vi "SEM Scan Parameter Coerce.vi"(6 "X full scale (V)":dbl, 7 "AI upper limit":dbl=100000000.0, 8 "SEM Status":T3={"AO SampClk.MaxRate"=100000000.0, "AI SampClk.MaxRate"=100000000.0, "AO rate"=10000000.0, "Scan speed"=4, "Detector #"=1, "X min (V)"=-10.0, "X max (V)"=10.0, "X min index"=0, "X max index"=1023, "AO multiline"=512, "Decimating factor"=2, "AvailSampPerChan"=0, "AO scan line"=0, "Total pixels recorded"=0, "Lines scanned"=0, "Scan time (m)"=0.0, "Scan time (s)"=4.15236096, "Remaining time (m)"=0, "Remaining time (s)"=0, "Specimen I (nA)"=0.0, "Frame"=1, "X tile"=1, "Y tile"=1} {"Frame" min=1 step=1; "Y tile" min=1; "X tile" min=1; "Specimen I (nA)" format="%.2g"; "AvailSampPerChan" scale=0.0..32000000.0; "Scan time (s)" format="%.3f"; "Total pixels recorded" scale=-1.0..37748736.0; "Scan speed" scale=1.0..15.0; "AO rate" format="%#_3e"}, 9 "SEM Options":T2={"GetInfo"=TRUE, "Set Det A para"=TRUE, "Set WD"=FALSE, "Set Mag"=TRUE, "Set stig"=FALSE, "Set aln"=FALSE, "Display"=TRUE, "Save"=TRUE, "8-bit"=TRUE, "Detector A"=TRUE, "Detector B"=FALSE, "Detector C"=FALSE, "Detector D"=FALSE, "Inverse A"=FALSE, "Inverse B"=FALSE, "Inverse C"=FALSE, "Inverse D"=FALSE, "Inverse PNG"=TRUE, "Freeze"=TRUE, "PNG only"=FALSE, "Upload"=FALSE, "Delete after upload"=FALSE}, 10 "SEM Scan Parameters":T1={"X size (um)"=20.0, "Y size (um)"=20.0, "X center (um)"=0.0, "Y center (um)"=0.0, "X size (V)"=6.190428211586902, "X size auto"=TRUE, "X stig"=[[0.0]], "Y stig"=[[0.0]], "X aln"=[[0.0]], "Y aln"=[[0.0]], "Scan rate (Hz)"=10000000, "Oversampling"=5, "Oversampling auto"=TRUE, "Frame line rampdown ratio"=0.1, "Pixel size (nm)"=10.0, "WD (mm)"=[[3.0]], "X tiles"=1, "Y tiles"=1, "Overlap (um)"=1.0, "Interlaced"=TRUE, "dX (um)"=[0.0], "dY (um)"=[0.0], "Frames"=1} {"dY (um)" format="%.1f"; "dX (um)" format="%.1f"; "Frames" min=1 step=1; "WD (mm)" format="%.1f"; "Y aln" format="%.1f"; "X aln" format="%.1f"; "Y stig" format="%.1f"; "X stig" format="%.1f"; "Overlap (um)" min=0; "Y tiles" min=1; "X tiles" min=1; "X size (um)" format="%.2f"; "Y size (um)" format="%.2f"; "Frame line rampdown ratio" min=0 max=1 step=0.05 format="%.2g"; "X center (um)" step=1.0 format="%.2f"; "Y center (um)" step=1.0 format="%.2f"; "X size (V)" format="%_4g"; "Scan rate (Hz)" max=4000000 step=100000 format="%.2e"}, 11 "Hardware Configuration":T4={"SEM X coil"="SEM-X", "SEM Y coil"="SEM-Y", "FIB X coil"="FIB/ao0", "FIB Y coil"="FIB/ao1", "FIB Detector"="FIB/ai1", "SEM Detectors"="Detectors", "Det min (V)"=-10.0, "Det max (V)"=10.0, "Eanable COM"=TRUE, "COM port"="COM1", "FIB Beam blank"="FIB/port0/line0", "FIB Ext Scan"="FIB/port0/line1", "Det. FIB-NI auto switch"="FIB/port0/line2", "Post #1up"="Log/ao0", "Post #1down"="Log/ao1", "Post #2up"="Log/ao2", "Post #2down"="Log/ao3", "Machine Type"=0, "FIB Faraday Cup"="FIB/ai3", "Configuration file"=path "D:/3D FIB-SEM Files/Feiss.ini", "SEM Max FOV (um)"=198.5, "Machine ID"="Feiss2/Merlin-4238", "Save config file"=FALSE, "Temperature port"="COM3", "Brightness A"=30.0, "Contrast A"=25.0, "Detector B name"="ESB", "Brightness B"=50.0, "Contrast B"=30.0, "Logging Device"="Log"} {"Machine Type" items=["Feiss", "NVision", "Jeiss"]}) -> (1 "Coerced SEM Scan Parameters":T1={"X size (um)"=20.0, "Y size (um)"=20.0, "X center (um)"=0.0, "Y center (um)"=0.0, "X size (V)"=6.190428211586902, "X size auto"=TRUE, "X stig"=[[0.0]], "Y stig"=[[0.0]], "X aln"=[[0.0]], "Y aln"=[[0.0]], "Scan rate (Hz)"=10000000, "Oversampling"=5, "Oversampling auto"=TRUE, "Frame line rampdown ratio"=0.1, "Pixel size (nm)"=10.0, "WD (mm)"=[[3.0]], "X tiles"=1, "Y tiles"=1, "Overlap (um)"=1.0, "Interlaced"=TRUE, "dX (um)"=[0.0], "dY (um)"=[0.0], "Frames"=1} {"dY (um)" format="%.1f"; "dX (um)" format="%.1f"; "Frames" min=1 step=1; "WD (mm)" format="%.1f"; "Y aln" format="%.1f"; "X aln" format="%.1f"; "Y stig" format="%.1f"; "X stig" format="%.1f"; "Overlap (um)" min=0; "Y tiles" min=1; "X tiles" min=1; "X size (um)" format="%.2f"; "Y size (um)" format="%.2f"; "Frame line rampdown ratio" min=0 max=1 step=0.05 format="%.2g"; "X center (um)" step=1.0 format="%.2f"; "Y center (um)" step=1.0 format="%.2f"; "X size (V)" format="%_4g"; "Scan rate (Hz)" max=4000000 step=100000 format="%.2e"}, 2 "SEM FOV":dbl=198.5, 3 "Detector number":i16)   [LabVIEW 2018]
panel:
  # "Det"
  # "after"
  # "Hz"
  # "Scanning time"
  # "m"
  # "s"
  # "Remaining time"
  # "m"
  # "s"
  # "Detector"
  # "Brightness & Contrast (%)"
  # "A       InLens"
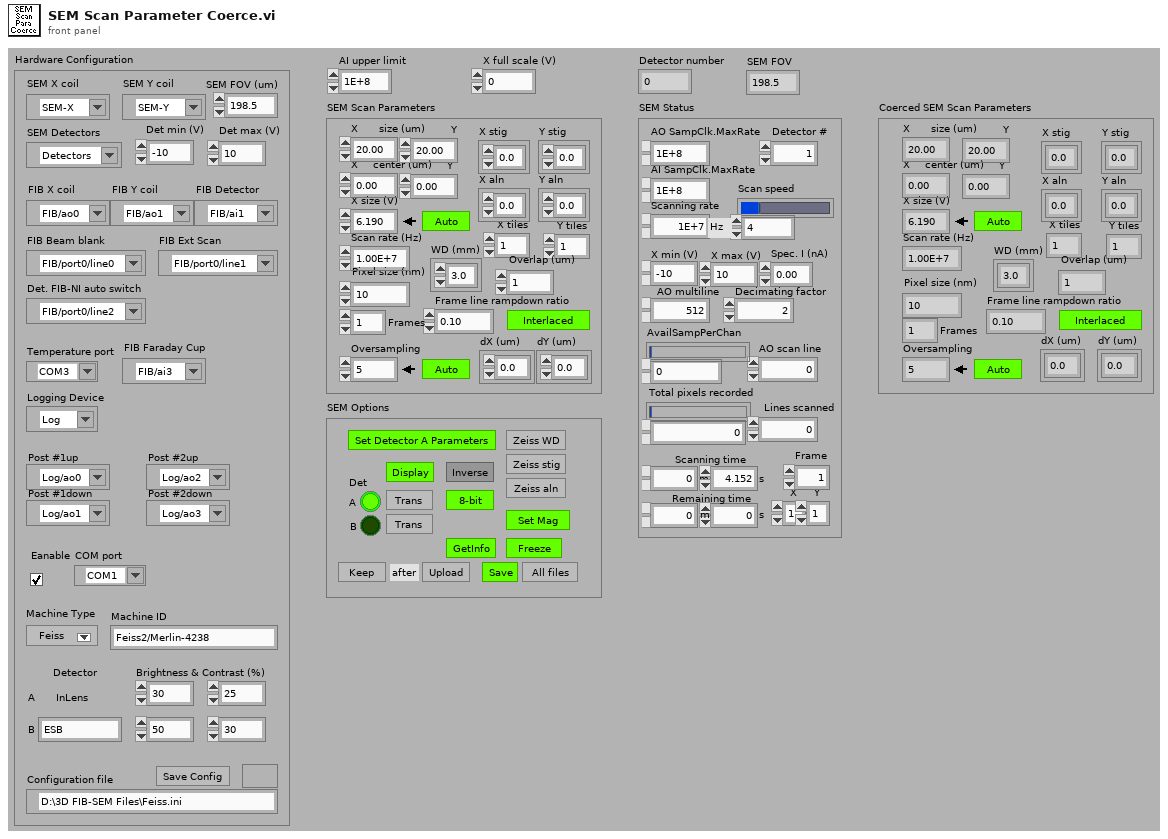
[diagram p1: front panel]
types:
  T1 = cluster{"X size (um)":sgl, "Y size (um)":sgl, "X center (um)":dbl, "Y center (um)":dbl, "X size (V)":dbl, "X size auto":bool, "X stig":sgl[][], "Y stig":sgl[][], "X aln":sgl[][], "Y aln":sgl[][], "Scan rate (Hz)":u32, "Oversampling":u32, "Oversampling auto":bool, "Frame line rampdown ratio":sgl, "Pixel size (nm)":sgl, "WD (mm)":sgl[][], "X tiles":u8, "Y tiles":u8, "Overlap (um)":sgl, "Interlaced":bool, "dX (um)":sgl[], "dY (um)":sgl[], "Frames":u8}
  T2 = cluster{"GetInfo":bool, "Set Det A para":bool, "Set WD":bool, "Set Mag":bool, "Set stig":bool, "Set aln":bool, "Display":bool, "Save":bool, "8-bit":bool, "Detector A":bool, "Detector B":bool, "Detector C":bool, "Detector D":bool, "Inverse A":bool, "Inverse B":bool, "Inverse C":bool, "Inverse D":bool, "Inverse PNG":bool, "Freeze":bool, "PNG only":bool, "Upload":bool, "Delete after upload":bool}
  T3 = cluster{"AO SampClk.MaxRate":dbl, "AI SampClk.MaxRate":dbl, "AO rate":dbl, "Scan speed":u8, "Detector #":u8, "X min (V)":dbl, "X max (V)":dbl, "X min index":i32, "X max index":i32, "AO multiline":u32, "Decimating factor":u16, "AvailSampPerChan":u32, "AO scan line":u32, "Total pixels recorded":i32, "Lines scanned":i32, "Scan time (m)":dbl, "Scan time (s)":dbl, "Remaining time (m)":u16, "Remaining time (s)":u8, "Specimen I (nA)":sgl, "Frame":u8, "X tile":u8, "Y tile":u8}
  T4 = cluster{"SEM X coil":refnum<k15>, "SEM Y coil":refnum<k15>, "FIB X coil":tag, "FIB Y coil":tag, "FIB Detector":tag, "SEM Detectors":refnum<k15>, "Det min (V)":dbl, "Det max (V)":dbl, "Eanable COM":bool, "COM port":refnum<visa-resource-name>, "FIB Beam blank":tag, "FIB Ext Scan":tag, "Det. FIB-NI auto switch":tag, "Post #1up":tag, "Post #1down":tag, "Post #2up":tag, "Post #2down":tag, "Machine Type":u8, "FIB Faraday Cup":tag, "Configuration file":path, "SEM Max FOV (um)":dbl, "Machine ID":string, "Save config file":bool, "Temperature port":refnum<visa-resource-name>, "Brightness A":dbl, "Contrast A":dbl, "Detector B name":string, "Brightness B":dbl, "Contrast B":dbl, "Logging Device":tag}
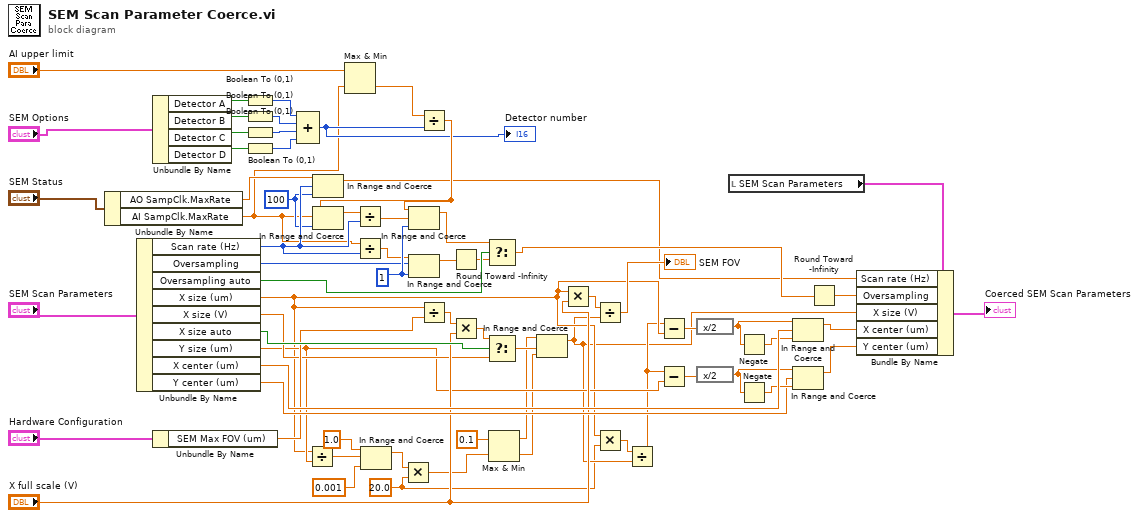
[diagram p0: block diagram]
diagram:
  w1 = 20.0 ("upper limit")
  w51 = u8 1 ("lower limit")
  w43 = u32 100 ("lower limit")
  n1 = Unbundle By Name("SEM Status") -> ("AO SampClk.MaxRate"=w39:dbl, "AI SampClk.MaxRate"=w24:dbl)
  n2 = Unbundle By Name("SEM Scan Parameters") -> ("Scan rate (Hz)"=w46:u32, "Oversampling"=w38:u32, "Oversampling auto"=w45:bool, "X size (um)"=w4:sgl, "X size (V)"=w15:dbl, "X size auto"=w54:bool, "Y size (um)"=w11:sgl, "X center (um)"=w67:dbl, "Y center (um)"=w57:dbl)
  n3 = Unbundle By Name("SEM Options") -> ("Detector A"=w30:bool, "Detector B"=w34:bool, "Detector C"=w35:bool, "Detector D"=w36:bool)
  n4 = Unbundle By Name("Hardware Configuration") -> ("SEM Max FOV (um)"=w53:dbl)
  n5 = Boolean To (0,1)(Boolean=w30) -> (0, 1=w29:i16)
  n6 = Boolean To (0,1)(Boolean=w34) -> (0, 1=w28:i16)
  n7 = Boolean To (0,1)(Boolean=w35) -> (0, 1=w33:i16)
  n8 = Boolean To (0,1)(Boolean=w36) -> (0, 1=w32:i16)
  n9 = Compound Arithmetic op=ADD(w29, w28, w33, w32) -> (w44:i16)
  "Detector number" <- w44
  n10 = Divide(x=w4, y=w11) -> (x/y=w22:sgl)
  n11 = In Range and Coerce(upper limit=w39, x=w46, lower limit=w43) -> (coerced(x)=w37:dbl)  [unwired: 1 out]
  n12 = Max & Min(x="AI upper limit", y=w24) -> (min(x,y)=w23:dbl)  [unwired: 1 out]
  n13 = Divide(x=w24, y=w46) -> (x/y=w47:dbl)
  n14 = In Range and Coerce(upper limit=1.0, x=w22, lower limit=0.001) -> (coerced(x)=w18:dbl)  [unwired: 1 out]
  n15 = Multiply(x=w18, y=w1) -> (x*y=w14:dbl)
  n16 = In Range and Coerce(upper limit=w47, x=w38, lower limit=w51) -> (coerced(x)=w48:dbl)  [unwired: 1 out]
  n17 = Divide(x=w23, y=w44) -> (x/y=w52:dbl)
  n18 = In Range and Coerce(upper limit=w52, x=w24, lower limit=w43) -> (coerced(x)=w42:dbl)  [unwired: 1 out]
  n19 = Divide(x=w42, y=w46) -> (x/y=w50:dbl)
  n20 = In Range and Coerce(upper limit=w52, x=w50, lower limit=w51) -> (coerced(x)=w49:dbl)  [unwired: 1 out]
  n21 = Divide(x=w4, y=w53) -> (x/y=w55:dbl)
  n22 = Round Toward -Infinity(1:w48) -> (0:w41:dbl)
  n23 = Multiply(x=w55, y="X full scale (V)") -> (x*y=w17:dbl)
  n24 = Select(t=w49, s=w45, f=w41) -> (s? t:f=w40:dbl)
  n25 = Select(t=w17, s=w54, f=w15) -> (s? t:f=w16:dbl)
  n26 = Max & Min(x=0.1 ("upper limit"), y=w14) -> (max(x,y)=w7:dbl, min(x,y)=w6:dbl)
  n27 = In Range and Coerce(upper limit=w7, x=w16, lower limit=w6) -> (coerced(x)=w2:dbl)  [unwired: 1 out]
  n28 = Multiply(x=w4, y="X full scale (V)") -> (x*y=w59:dbl)
  n29 = Divide(x=w59, y=w2) -> (x/y=→"SEM FOV":dbl)
  n30 = Multiply(x=w4, y=w1) -> (x*y=w5:dbl)
  n31 = Divide(x=w5, y=w2) -> (x/y=w3:dbl)
  n32 = Subtract(x=w3, y=w4) -> (x-y=w63:dbl)
  n33 = Subtract(x=w3, y=w11) -> (x-y=w56:dbl)
  n34 = expression code="x/2"(w63) -> (w61:dbl)
  n35 = expression code="x/2"(w56) -> (w60:dbl)
  n36 = local read "SEM Scan Parameters"() -> (w10:T1)
  n37 = Negate(x=w61) -> (-x=w62:dbl)
  n38 = Negate(x=w60) -> (-x=w64:dbl)
  n39 = In Range and Coerce(upper limit=w61, x=w67, lower limit=w62) -> (coerced(x)=w66:dbl)  [unwired: 1 out]
  n40 = In Range and Coerce(upper limit=w60, x=w57, lower limit=w64) -> (coerced(x)=w58:dbl)  [unwired: 1 out]
  n41 = Round Toward -Infinity(1:w40) -> (0:w8:dbl)
  n42 = Bundle By Name(cluster=w10, "Scan rate (Hz)"=w37, "Oversampling"=w8, "X size (V)"=w2, "X center (um)"=w66, "Y center (um)"=w58) -> (→"Coerced SEM Scan Parameters":T1)
